vi "SingleElementsArray To Data_csm.vi"(7 "Pototype":variant, 8 "error in (no error)":errorcluster, 11 "DataElementArray":variant[](array[variant])) -> (0 "error out":errorcluster, 3 "Cluster":variant)   [LabVIEW 2017, in "API String Arguments Support.lvlib"]
doc: "This VI converts a DataELementArray to a Cluster."
uses:
  API String Arguments Support.lvlib
  <userlib>/_NEVSTOP/Communicable State Machine(CSM)/Communicable State Machine.lvlib
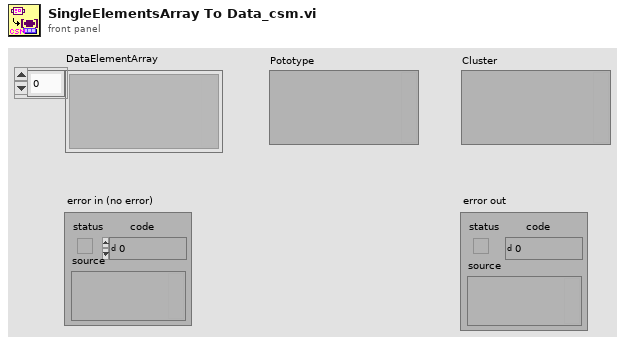
[diagram p1: front panel]
types:
  T1 = enum8{"<Null>", "I8", "I16", "I32", "I64", "U8", "U16", "U32", "U64", "SGL", "DBL", "EXT", "CSG", "CDB", "CXT", "0x0F", "0x10", "0x11", "0x12", "0x13", "0x14", "Enum U8", "Enum U16", "Enum U32", "Enum U64", "SGL PQ", "DBL PQ", "EXT PQ", "CSG PQ", "CDB PQ", "CXT PQ", "0x1F", "0x20", "Boolean", "0x22", "0x23", "0x24", "0x25", "0x26", "0x27", "0x28", "0x29", "0x2A", "0x2B", "0x2C", "0x2D", "0x2E", "0x2F", "String", "0x31", "Path", "Pict", "0x34", "0x35", "0x36", "DAQ", "0x38", "0x39", "0x3A", "0x3B", "0x3C", "0x3D", "0x3E", "0x3F", "Array", "0x41", "0x42", "0x43", "0x44", "0x45", "0x46", "0x47", "0x48", "0x49", "0x4A", "0x4B", "0x4C", "0x4D", "0x4E", "0x4F", "Cluster", "0x51", "0x52", "Variant", "Waveform", "0x55", "0x56", "0x57", "0x58", "0x59", "0x5A", "0x5B", "0x5C", "0x5D", "0x5E", "Fixed Point", "0x60", "0x61", "0x62", "0x63", "0x64", "0x65", "0x66", "0x67", "0x68", "0x69", "0x6A", "0x6B", "0x6C", "0x6D", "0x6E", "0x6F", "Refnum", "0x71", "0x72", "Set Collection", "Map Collection"}
  T2 = cluster{"length":u16, "private":u8, "type":enum8{"<Null>", "I8", "I16", "I32", "I64", "U8", "U16", "U32", "U64", "SGL", "DBL", "EXT", "CSG", "CDB", "CXT", "0x0F", "0x10", "0x11", "0x12", "0x13", "0x14", "Enum U8", "Enum U16", "Enum U32", "Enum U64", "SGL PQ", "DBL PQ", "EXT PQ", "CSG PQ", "CDB PQ", "CXT PQ", "0x1F", "0x20", "Boolean", "0x22", "0x23", "0x24", "0x25", "0x26", "0x27", "0x28", "0x29", "0x2A", "0x2B", "0x2C", "0x2D", "0x2E", "0x2F", "String", "0x31", "Path", "Pict", "0x34", "0x35", "0x36", "DAQ", "0x38", "0x39", "0x3A", "0x3B", "0x3C", "0x3D", "0x3E", "0x3F", "Array", "0x41", "0x42", "0x43", "0x44", "0x45", "0x46", "0x47", "0x48", "0x49", "0x4A", "0x4B", "0x4C", "0x4D", "0x4E", "0x4F", "Cluster", "0x51", "0x52", "Variant", "Waveform", "0x55", "0x56", "0x57", "0x58", "0x59", "0x5A", "0x5B", "0x5C", "0x5D", "0x5E", "Fixed Point", "0x60", "0x61", "0x62", "0x63", "0x64", "0x65", "0x66", "0x67", "0x68", "0x69", "0x6A", "0x6B", "0x6C", "0x6D", "0x6E", "0x6F", "Refnum", "0x71", "0x72", "Set Collection", "Map Collection"}, "# elements":u16}
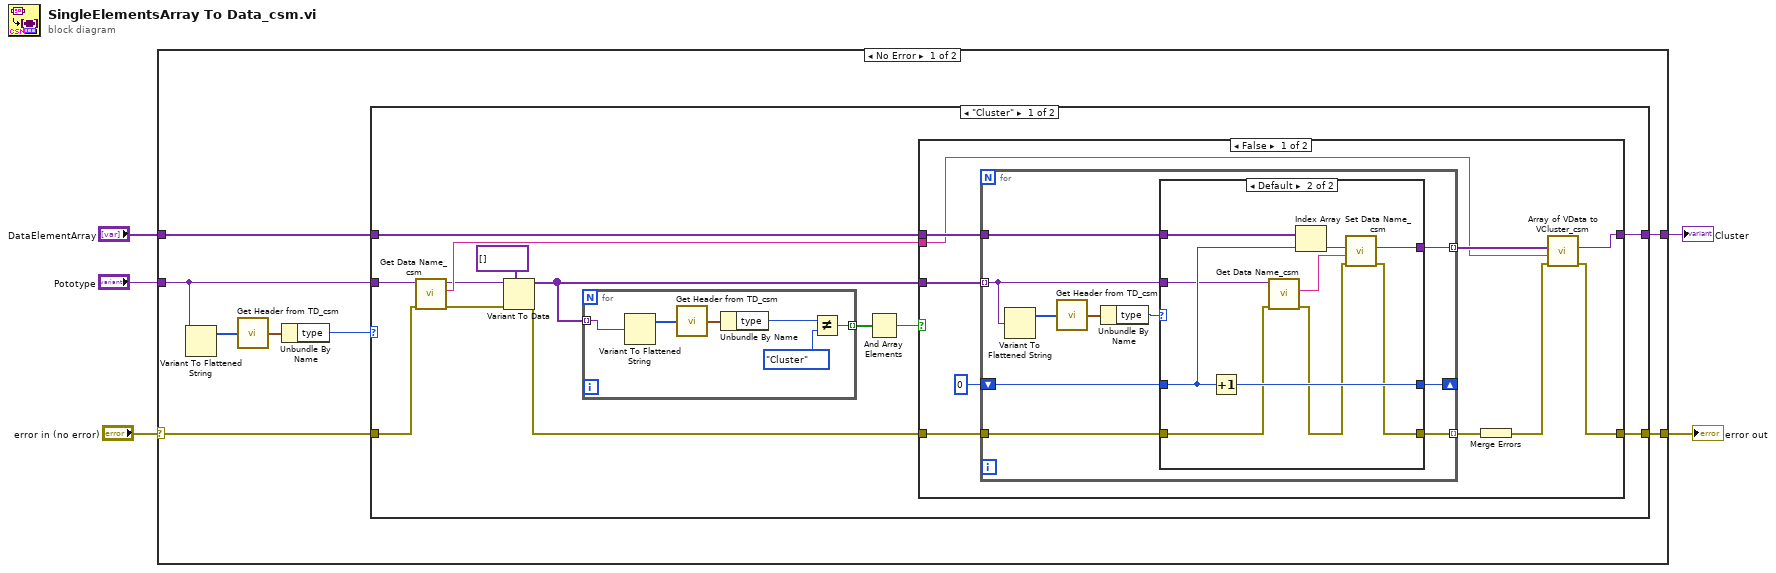
[diagram p0: block diagram]
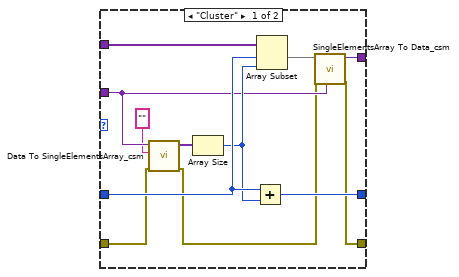
[diagram p2: hidden frame]
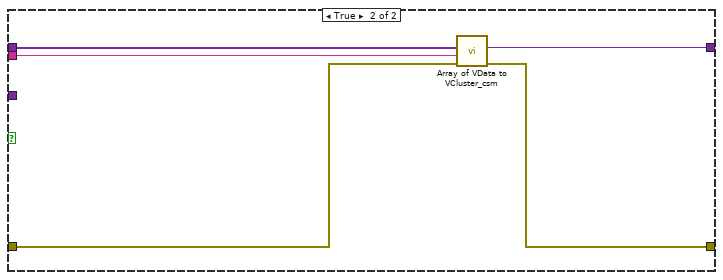
[diagram p3: hidden frame]
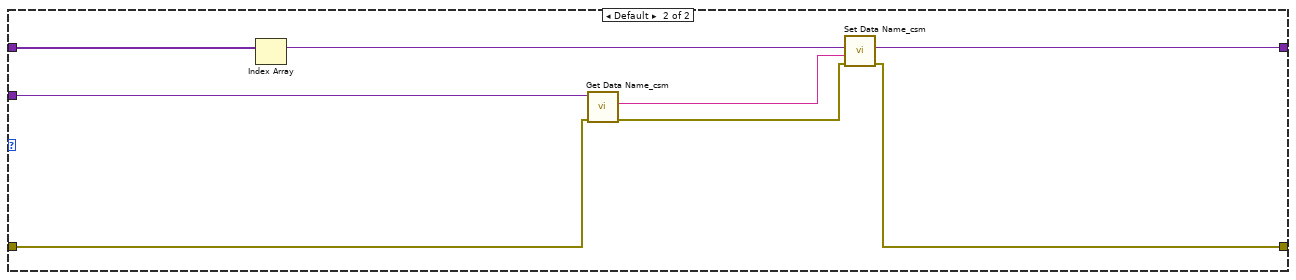
[diagram p4: hidden frame]
diagram:
  n1 = case shown="No Error" "error in (no error)" {
    selector: "error in (no error)" -> [w11 w88]
    tunnel: "DataElementArray" -> [w13 _]
    tunnel: [w12 w89] -> w4
    tunnel: [w10 w88] -> w2
    tunnel: "Pototype" -> [w7 w89]
    frame No Error {
      n2 = Variant To Flattened String(Variant=w7) -> (1:w9:i16[])  [unwired: 1 out]
      n3 = call <userlib>:"Get Header from TD_csm.vi"("Type Descriptor"=w9) -> ("Type Descriptor Header"=w8:T2)
      n4 = Unbundle By Name(w8) -> ("type"=w6:T1)
      n5 = case shown="\"Cluster\"" w6 {
        tunnel: w7 -> [w26 w84]
        tunnel: w13 -> [w23 w87]
        tunnel: [w22 w85] -> w12
        tunnel: w11 -> [w19 w82]
        tunnel: [w21 w80] -> w10
        frame "Cluster" {
          n6 = call <userlib>:"Get Data Name_csm.vi"("error in (no error)"=w19, "Data"=w26) -> ("error out"=w15:errorcluster, "Data Name"=w20:string, "Data dup"=w16:variant)  [unwired: 7 in]
          n7 = Variant To Data(error in=w15, type=variant[] [] ("Array"), Variant=w16) -> (data=w17:variant[], error out=w14:errorcluster)
          n8 = for {
            tunnel: w17 -> [w74] mode=indexing
            tunnel: [w78] -> w25 mode=indexing
            n9 = Variant To Flattened String(Variant=w74) -> (1:w77:i16[])  [unwired: 1 out]
            n10 = call <userlib>:"Get Header from TD_csm.vi"("Type Descriptor"=w77) -> ("Type Descriptor Header"=w76:T2)
            n11 = Unbundle By Name(w76) -> ("type"=w75:T1)
            n12 = Not Equal?(x=w75, y=T1."Cluster") -> (x != y?=w78:bool)
          }
          n13 = And Array Elements(Boolean array=w25) -> (logical AND=w24:bool)
          n14 = case shown="False" w24 {
            tunnel: w23 -> [w32 w73]
            tunnel: [w35 w72] -> w22
            tunnel: w17 -> [w36 _]
            tunnel: w14 -> [w31 w71]
            tunnel: [w27 w70] -> w21
            tunnel: w20 -> [w29 w69]
            frame False {
              n15 = for {
                tunnel: w36 -> [w38] mode=indexing
                tunnel: [w46] -> w34 mode=indexing
                shift-right: [w43] -> _
                shift-left: 0 -> [w44]
                tunnel: w32 -> [w45]
                tunnel: w31 -> [w42]
                tunnel: [w41] -> w30 mode=indexing
                n16 = Variant To Flattened String(Variant=w38) -> (1:w40:i16[])  [unwired: 1 out]
                n17 = call <userlib>:"Get Header from TD_csm.vi"("Type Descriptor"=w40) -> ("Type Descriptor Header"=w39:T2)
                n18 = Unbundle By Name(w39) -> ("type"=w37:T1)
                n19 = case shown="Default" w37 {
                  tunnel: w38 -> [w52 w61]
                  tunnel: [w58 w62] -> w46
                  tunnel: w45 -> [w57 w68]
                  tunnel: w44 -> [w56 w67]
                  tunnel: [w54 w66] -> w43
                  tunnel: w42 -> [w49 w60]
                  tunnel: [w47 w59] -> w41
                  frame "Cluster" {
                    n20 = call "Data To SingleElementsArray_csm.vi"("error in (no error)"=w49, "parentUrl"="", "Cluster"=w52) -> ("error out"=w48:errorcluster, "DataElementArray"=w50:variant[])  [unwired: 6 in, 1 out]
                    n21 = Array Size(array=w50) -> (size(s)=w55:i32)
                    n22 = Add(x=w56, y=w55) -> (x+y=w54:i32)
                    n23 = Array Subset(array=w57, index=w56, length=w55) -> (w53:variant[])
                    n24 = call "SingleElementsArray To Data_csm.vi"("Pototype"=w52, "error in (no error)"=w48, "DataElementArray"=w53) -> ("error out"=w47:errorcluster, "Cluster"=w58:variant)  [unwired: 7 in]
                  }
                  frame Default {
                    n25 = Increment(x=w67) -> (x+1=w66:i32)
                    n26 = call <userlib>:"Get Data Name_csm.vi"("error in (no error)"=w60, "Data"=w61) -> ("error out"=w64:errorcluster, "Data Name"=w65:string)  [unwired: 7 in, 1 out]
                    n27 = Index Array(array=w68, index=w67) -> (element=w63:variant)
                    n28 = call <userlib>:"Set Data Name_csm.vi"("error in (no error)"=w64, "Data Name"=w65, "Data"=w63) -> ("error out"=w59:errorcluster, "Renamed Data"=w62:variant)  [unwired: 7 in]
                  }
                }
              }
              n29 = Merge Errors(w30) -> (w28:errorcluster)
              n30 = call <userlib>:"Array of VData to VCluster_csm.vi"("error in (no error)"=w28, "Cluster Name"=w29, "Array"=w34) -> ("error out"=w27:errorcluster, "VCluster"=w35:variant)  [unwired: 7 in]
            }
            frame True {
              n31 = call <userlib>:"Array of VData to VCluster_csm.vi"("error in (no error)"=w71, "Cluster Name"=w69, "Array"=w73) -> ("error out"=w70:errorcluster, "VCluster"=w72:variant)  [unwired: 7 in]
            }
          }
        }
        frame Default {
          n32 = Index Array(array=w87) -> (element=w86:variant)  [unwired: 1 in]
          n33 = call <userlib>:"Get Data Name_csm.vi"("error in (no error)"=w82, "Data"=w84) -> ("error out"=w81:errorcluster, "Data Name"=w83:string)  [unwired: 7 in, 1 out]
          n34 = call <userlib>:"Set Data Name_csm.vi"("error in (no error)"=w81, "Data Name"=w83, "Data"=w86) -> ("error out"=w80:errorcluster, "Renamed Data"=w85:variant)  [unwired: 7 in]
        }
      }
    }
    frame Error {
    }
  }
  "error out" <- w2
  "Cluster" <- w4
